vi "Init_ReqNum.vi"(8 "error in (no error)":errorcluster, 11 "UserID":string) -> (0 "error out":errorcluster, 2 "ReqID":string)   [LabVIEW 2017, in "ArduinoRemote.lvlib"]
uses:
  ArduinoRemote.lvlib
panel:
  out "date/time string":string
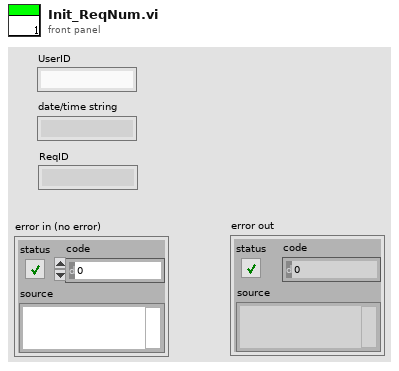
[diagram p1: front panel]
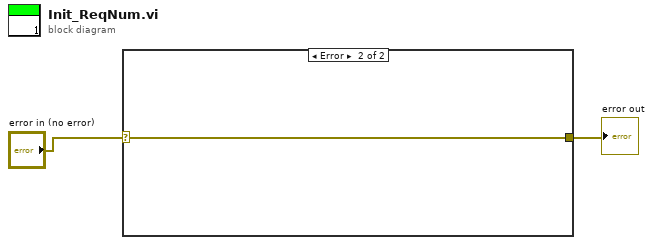
[diagram p0: block diagram]
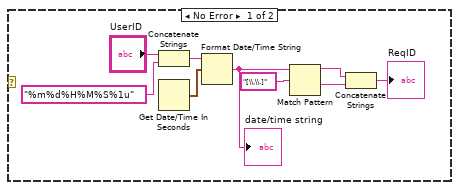
[diagram p2: hidden frame]
diagram:
  n1 = case shown="Error" "error in (no error)" {
    selector: "error in (no error)" -> [_ w12]
    tunnel: [_ w12] -> w1
    frame No Error {
      n2 = Concatenate Strings("UserID", "%m%d%H%M%S%1u" ("time format string (%c)")) -> (w3:string)
      n3 = Get Date/Time In Seconds() -> (seconds since 1Jan1904=w6:timestamp)
      n4 = Format Date/Time String(time format string (%c)=w3, seconds (now)=w6) -> (date/time string=w7:string)  [unwired: 1 in]
      "date/time string" <- w7
      n5 = Match Pattern(string=w7, regular expression="[\\,\\.]") -> (before substring=w9:string, after substring=w10:string)  [unwired: 1 in, 2 out]
      n6 = Concatenate Strings(w9, w10) -> (→"ReqID":string)
    }
    frame Error {
    }
  }
  "error out" <- w1
